vi "E727_SingleChannelMove.vi"() -> ()   [LabVIEW 2022 SP3]
doc: "This VI demonstrates how to initialize an E-727 system, how to move one connected axis and how to query for the position value of this axis. \nIn this example the E-727 is connected through COM port 1 with baudrate 115200. The VI runs E727_Configuration_Setup.vi with these specified settings, moves the first connected axis relative to its current position and reads the position of this axis. The diagram shows how to combine the driver VIs for these tasks. \nWarning: Before running this VI, modify the \"Interface\" and \"RS232 settings\" (or TCP/IP settings or USB settings ) to reflect your configuration. The predefined settings provided with the VI probably do not match your system."
panel:
  out "StageRunning 3":bool
  out "StageRunning 2":bool
  in  "Target AbsolutePosition (um)":dbl[](array[numeric]) format="%.6f"
  out "Progress":dbl(slide) scale=0.0..100.0
  out "Loop counter":dbl
  in  "Type of Motion":bool
  in  "Map size":i32
  in  "Relative Resolution (um)":dbl[](array[numeric]) format="%.6f"
  out "Initial position":dbl[](array[numeric]) format="%.6f"
  in  "error in":errorcluster
  out "StageRunning":bool
  in  "StageOn/Off":bool
  in  "Start Move":bool
  out "Pre-move position":dbl[](array[numeric]) format="%.6f"
  in  "stop":bool
  out "error out":errorcluster
  out "Current position":dbl[](array[numeric]) format="%.6f"
  # "This IV allows for user to perform Absolute positionsing or a NxN array relative move based on a resolution. \nInstructions\n1) Turn on Stage\n2) Select Absolute Motion or Relative Motion\n3) Fill out motion values depending on the selected motion"
  # "Y\nX"
  # "Absolute motion"
  # "Relative motion"
  # "Y\nX\nZ"
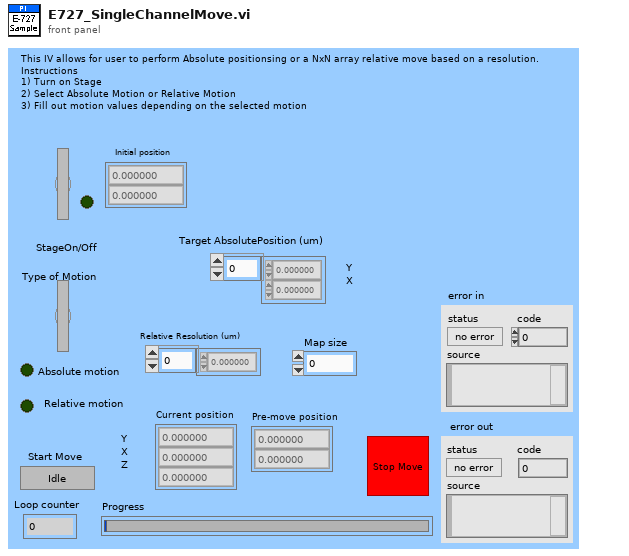
[diagram p1: front panel]
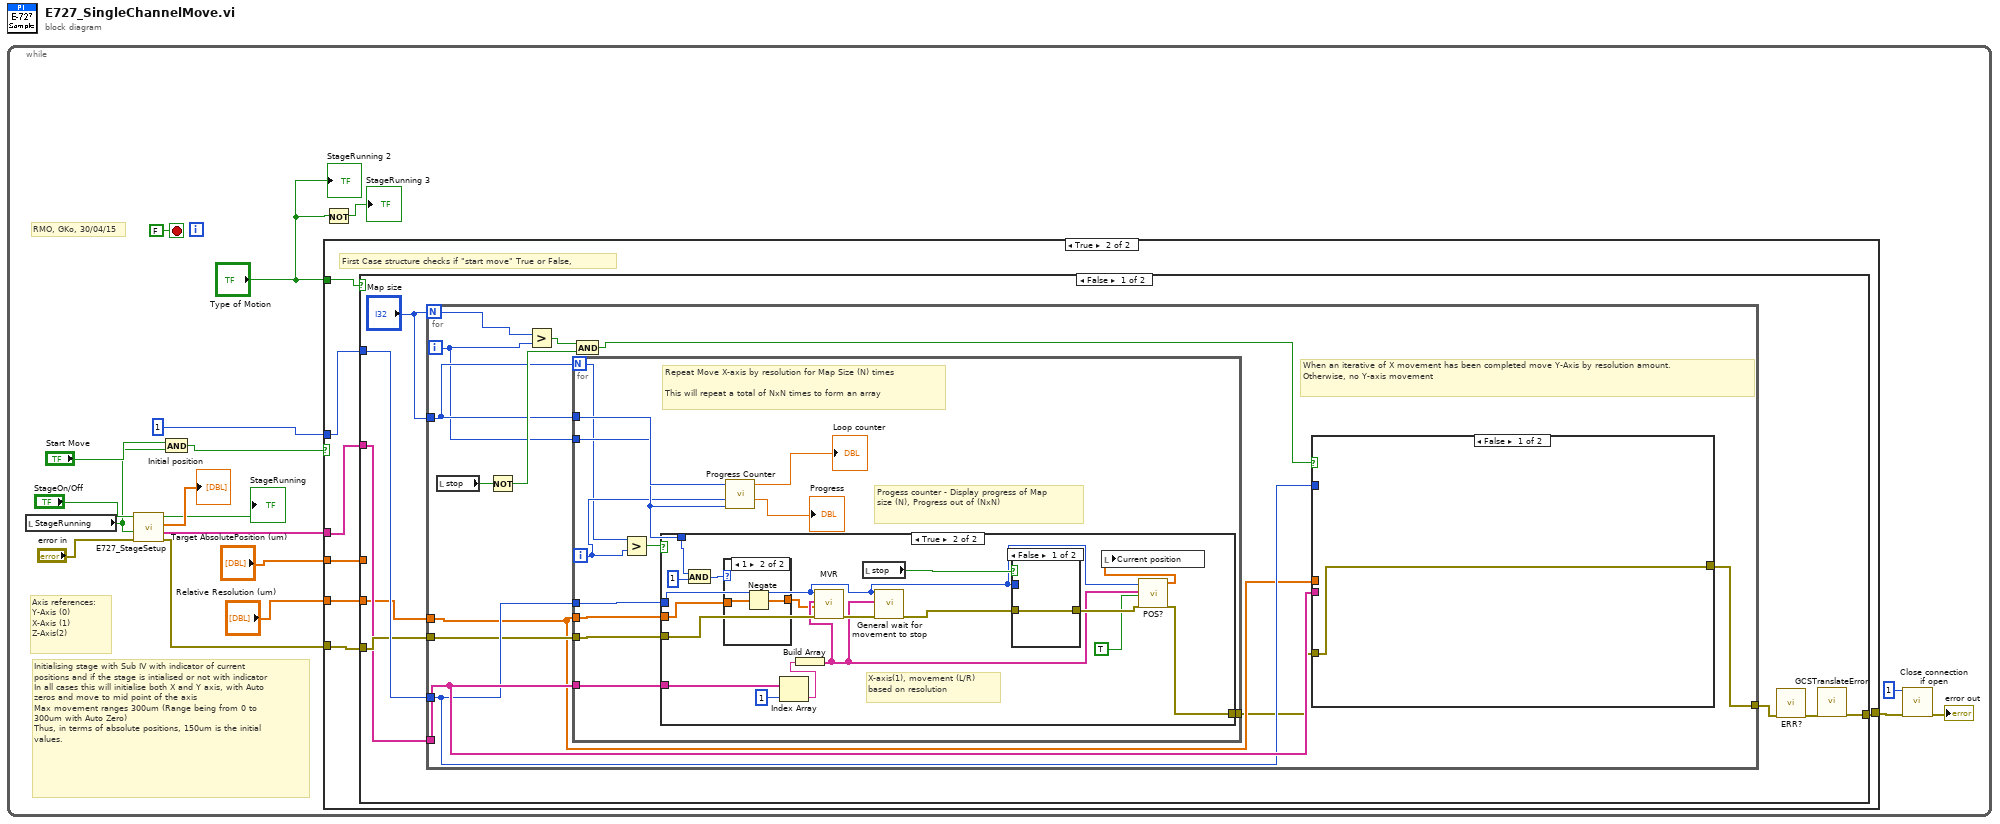
[diagram p0: block diagram]
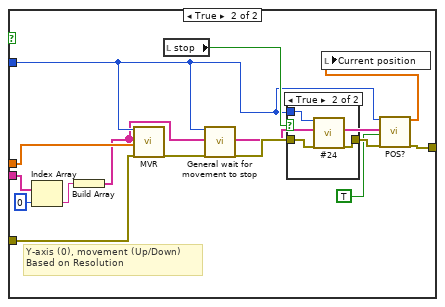
[diagram p3: hidden frame]
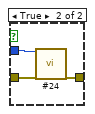
[diagram p7: hidden frame]
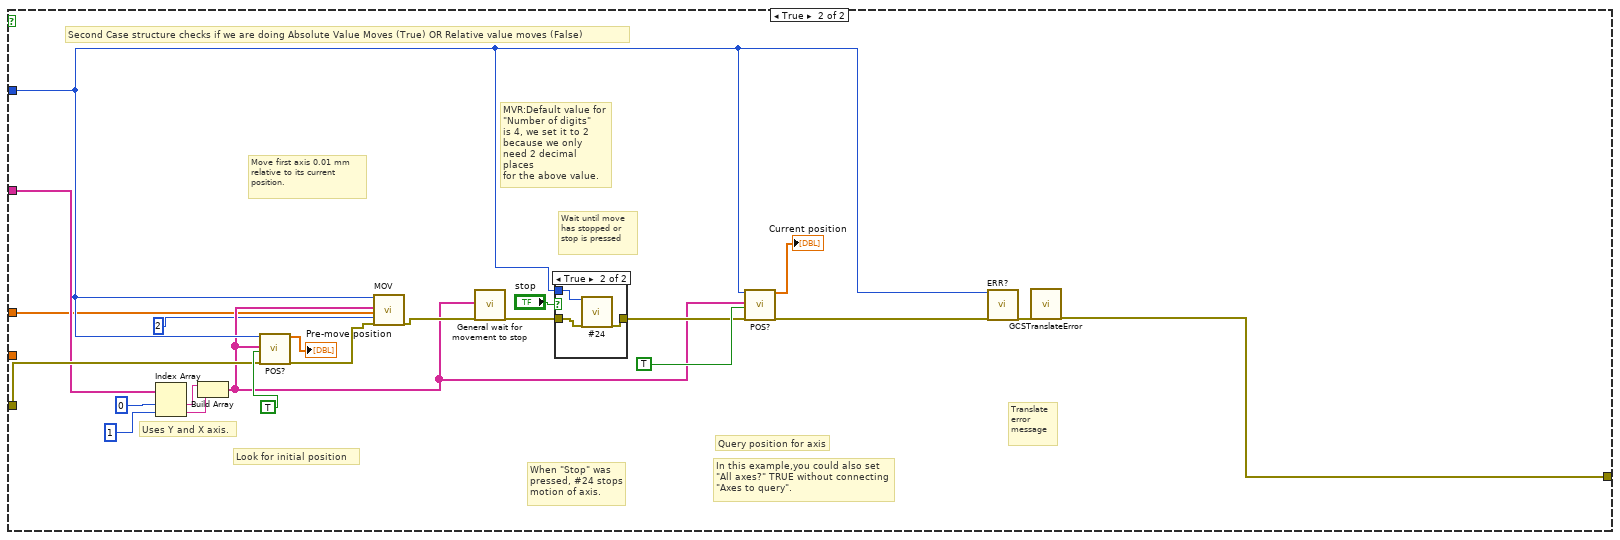
[diagram p8: hidden frame]
diagram:
  n1 = while {
    stop <- FALSE stop-if-true
    # "Axis references:\nY-Axis (0)\nX-Axis (1)\nZ-Axis(2)"
    # "Initialising stage with Sub IV with indicator of current positions and if the stage is intialised or not with indicator\nIn all cases this will initialise both X and Y axis, with Auto zeros and move to mid point of the axis \nMax movement ranges 300um (Range being from 0 to 300um with Auto Zero)\nThus, in terms of absolute positions, 150um is the initial values."
    # "RMO, GKo, 30/04/15"
    n2 = local read "StageRunning"() -> (w9:bool)
    n3 = call "E727_StageSetup.vi"("error in"="error in", "StageRunningIn"=w9, "StageOn/Off"="StageOn/Off") -> ("error out"=w8:errorcluster, "StageChannels"=w7:string[], "Current position"=→"Initial position":dbl[], "StageRunningOut"=→"StageRunning":bool)  [unwired: 5 in]
    n4 = And(x="Start Move", y=w9) -> (x .and. y?=w17:bool)
    n5 = case shown="True" w17 {
      tunnel: w7 -> [_ w23]
      tunnel: w8 -> [w19 w25]
      tunnel: [w19 w26] -> w13
      tunnel: 1 ("System no.") -> [_ w24]
      tunnel: "Relative Resolution (um)" -> [_ w22]
      tunnel: "Type of Motion" -> [_ w21]
      tunnel: "Target AbsolutePosition (um)" -> [_ w20]
      frame False {
      }
      frame True {
        # "First Case structure checks if \"start move\" True or False,"
        n6 = case shown="False" w21 {
          tunnel: [w29 w117] -> w26
          tunnel: w25 -> [w31 w115]
          tunnel: w24 -> [w32 w112]
          tunnel: w23 -> [w30 w113]
          tunnel: w22 -> [w28 _]
          tunnel: w20 -> [_ w105]
          frame False {
            n7 = for {
              N: "Map size" -> [w35]
              tunnel: "Map size" -> [w40]
              tunnel: w31 -> [w43]
              tunnel: w32 -> [w44]
              tunnel: w30 -> [w45]
              tunnel: [w38] -> w27
              tunnel: w28 -> [w42]
              i -> [w36]
              # "When an iterative of X movement has been completed move Y-Axis by resolution amount.\nOtherwise, no Y-axis movement"
              n8 = local read "stop"() -> (w46:bool)
              n9 = Not(x=w46) -> (.not. x?=w47:bool)
              n10 = Greater?(x=w35, y=w36) -> (0:w37:bool)
              n11 = for {
                N: w40 -> [w67]
                tunnel: w43 -> [w78]
                tunnel: w44 -> [w77]
                tunnel: w45 -> [w76]
                tunnel: w42 -> [w75]
                tunnel: w40 -> [w74]
                tunnel: w36 -> [w70]
                tunnel: [w71] -> w39
                i -> [w69]
                # "Repeat Move X-axis by resolution for Map Size (N) times\n\nThis will repeat a total of NxN times to form an array"
                # "Progess counter - Display progress of Map size (N), Progress out of (NxN)"
                n12 = Greater?(x=w67, y=w69) -> (0:w68:bool)
                n13 = case shown="True" w68 {
                  tunnel: w76 -> [_ w94]
                  tunnel: w78 -> [w79 w93]
                  tunnel: w77 -> [_ w89]
                  tunnel: w75 -> [_ w81]
                  tunnel: [w79 w87] -> w71
                  tunnel: w70 -> [_ w83]
                  frame False {
                  }
                  frame True {
                    # "X-axis(1), movement (L/R) based on resolution"
                    n14 = And(x=w83, y=1) -> (x .and. y?=w85:i32)
                    n15 = case shown="1" w85 {
                      tunnel: [w98 w99] -> w82
                      tunnel: w81 -> [w98 w100]
                      frame 0, Default {
                      }
                      frame 1 {
                        n16 = Negate(x=w100) -> (-x=w99:dbl[])
                      }
                    }
                    n17 = Index Array(array=w94, index=1) -> (element=w95:string)
                    n18 = Build Array(w95) -> (w88:string[])
                    n19 = call "MVR.vi"("System no."=w89, "Axes to move"=w88, "Position values"=w82, "error in"=w93) -> ("error out"=w97:errorcluster)  [unwired: 1 in, 14 out]
                    n20 = local read "stop"() -> (w90:bool)
                    n21 = call "General wait for movement to stop.vi"("System no."=w89, "Axes to wait for"=w88, "error in"=w97) -> ("error out"=w92:errorcluster)  [unwired: 5 in, 11 out]
                    n22 = case shown="False" w90 {
                      tunnel: w92 -> [w101 w104]
                      tunnel: [w101 w103] -> w91
                      tunnel: w89 -> [_ w102]
                      frame False {
                      }
                      frame True {
                        n23 = call "#24.vi"("System no."=w102, "error in"=w104) -> ("error out"=w103:errorcluster)  [unwired: 17 out]
                      }
                    }
                    n24 = call "POS?.vi"("System no."=w89, "Axes to query"=w88, "All axes?"=TRUE, "error in"=w91) -> ("Position"=w86:dbl[], "error out"=w87:errorcluster)  [unwired: 1 in, 13 out]
                    n25 = local write "Current position"(w86) -> ()
                  }
                }
                n26 = call "Progress Counter.vi"("y"=w70, "x"=w69, "Map size (Pixels)"=w74) -> ("Progress"=→"Progress":dbl, "Loop counter"=→"Loop counter":dbl)  [unwired: 7 in]
              }
              n27 = And(x=w37, y=w47) -> (x .and. y?=w41:bool)
              n28 = case shown="False" w41 {
                tunnel: w45 -> [_ w59]
                tunnel: w44 -> [_ w51]
                tunnel: w39 -> [w48 w58]
                tunnel: w42 -> [_ w55]
                tunnel: [w48 w53] -> w38
                frame False {
                }
                frame True {
                  # "Y-axis (0), movement (Up/Down)\nBased on Resolution"
                  n29 = Index Array(array=w59, index=0) -> (element=w61:string)
                  n30 = Build Array(w61) -> (w50:string[])
                  n31 = call "MVR.vi"("System no."=w51, "Axes to move"=w50, "Position values"=w55, "error in"=w58) -> ("error out"=w60:errorcluster)  [unwired: 1 in, 14 out]
                  n32 = local read "stop"() -> (w57:bool)
                  n33 = call "General wait for movement to stop.vi"("System no."=w51, "Axes to wait for"=w50, "error in"=w60) -> ("error out"=w56:errorcluster)  [unwired: 5 in, 11 out]
                  n34 = case shown="True" w57 {
                    tunnel: w56 -> [w63 w66]
                    tunnel: [w63 w65] -> w54
                    tunnel: w51 -> [_ w64]
                    frame False {
                    }
                    frame True {
                      n35 = call "#24.vi"("System no."=w64, "error in"=w66) -> ("error out"=w65:errorcluster)  [unwired: 17 out]
                    }
                  }
                  n36 = call "POS?.vi"("System no."=w51, "Axes to query"=w50, "All axes?"=TRUE, "error in"=w54) -> ("Position"=w52:dbl[], "error out"=w53:errorcluster)  [unwired: 1 in, 13 out]
                  n37 = local write "Current position"(w52) -> ()
                }
              }
            }
            n38 = call "ERR?.vi"("error in"=w27) -> ("error out"=w33:errorcluster)  [unwired: 1 in, 17 out]
            n39 = call "GCSTranslateError.vi"("error in"=w33) -> ("error out"=w29:errorcluster)  [unwired: 18 out]
          }
          frame True {
            # "Look for initial position"
            # "Second Case structure checks if we are doing Absolute Value Moves (True) OR Relative value moves (False)"
            # "Uses Y and X axis."
            # "When \"Stop\" was \npressed, #24 stops\nmotion of axis."
            # "Translate\nerror \nmessage"
            # "Wait until move\nhas stopped or\nstop is pressed"
            # "MVR:Default value for\n\"Number of digits\"\nis 4, we set it to 2\nbecause we only\nneed 2 decimal places\nfor the above value."
            # "Move first axis 0.01 mm\nrelative to its current\nposition."
            # "In this example,you could also set \n\"All axes?\" TRUE without connecting\n\"Axes to query\"."
            # "Query position for axis"
            n40 = Index Array(array=w113, index #1=0 ("index"), index #2=1 ("index")) -> (element #1=w119:string, element #2=w107:string)
            n41 = Build Array(w119, w107) -> (w109:string[])
            n42 = call "POS?.vi"("System no."=w112, "Axes to query"=w109, "All axes?"=TRUE, "error in"=w115) -> ("Position"=→"Pre-move position":dbl[], "error out"=w111:errorcluster)  [unwired: 1 in, 13 out]
            n43 = call "MOV.vi"("System no."=w112, "Axes to move"=w109, "Position values"=w105, "No.of digits"=i16 2, "error in"=w111) -> ("error out"=w110:errorcluster)  [unwired: 14 out]
            n44 = call "General wait for movement to stop.vi"("Axes to wait for"=w109, "error in"=w110) -> ("error out"=w125:errorcluster)  [unwired: 6 in, 11 out]
            n45 = case shown="True" "stop" {
              tunnel: w125 -> [w127 w130]
              tunnel: [w127 w129] -> w124
              tunnel: w112 -> [_ w128]
              frame False {
              }
              frame True {
                n46 = call "#24.vi"("System no."=w128, "error in"=w130) -> ("error out"=w129:errorcluster)  [unwired: 17 out]
              }
            }
            n47 = call "POS?.vi"("System no."=w112, "Axes to query"=w109, "All axes?"=TRUE, "error in"=w124) -> ("Position"=→"Current position":dbl[], "error out"=w122:errorcluster)  [unwired: 1 in, 13 out]
            n48 = call "ERR?.vi"("System no."=w112, "error in"=w122) -> ("error out"=w121:errorcluster)  [unwired: 17 out]
            n49 = call "GCSTranslateError.vi"("error in"=w121) -> ("error out"=w117:errorcluster)  [unwired: 18 out]
          }
        }
      }
    }
    n50 = Not(x="Type of Motion") -> (.not. x?=→"StageRunning 3":bool)
    n51 = call "Close connection if open.vi"("System no."=1, "error in"=w13) -> ("error out"=→"error out":errorcluster)  [unwired: 1 in, 16 out]
    "StageRunning 2" <- "Type of Motion"
  }
